vi "Dresden Edit Recipe(in).vi"() -> ()   [LabVIEW 2009] (continued)
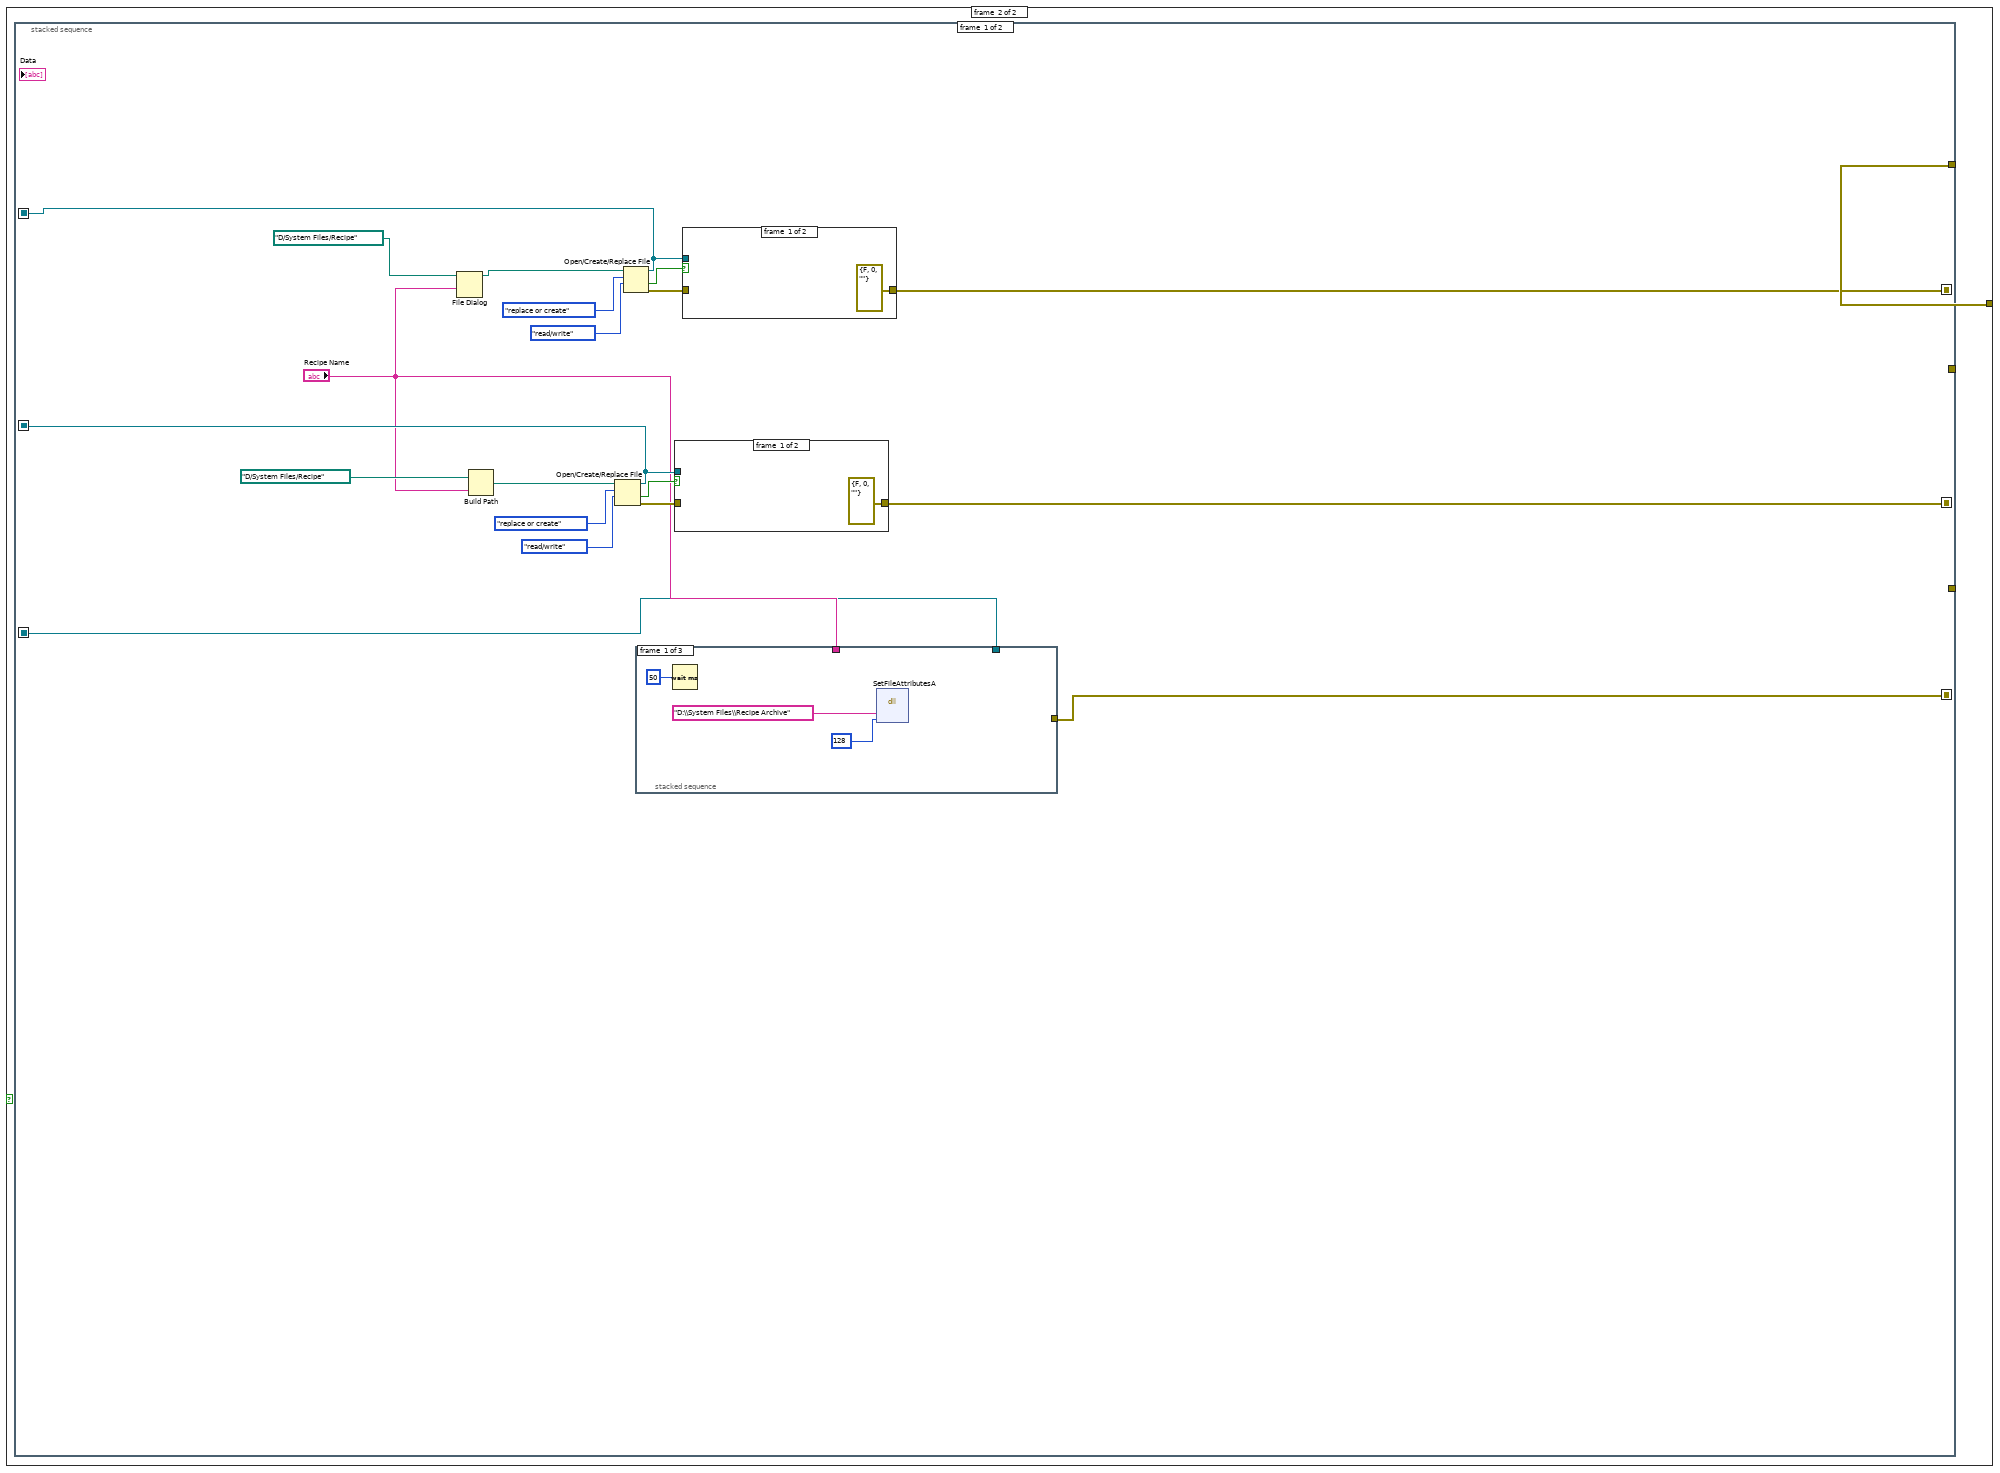
[diagram p2: hidden frame]
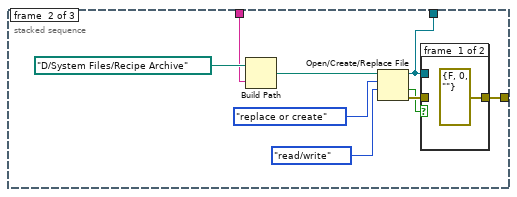
[diagram p3: hidden frame]
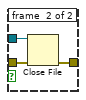
[diagram p4: hidden frame]
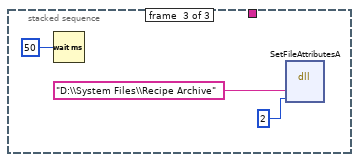
[diagram p5: hidden frame]
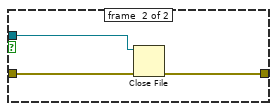
[diagram p6: hidden frame]
                }
                frame #1 {
                }
              }
              n2527 = Format Into String(format string="%s%s%s%s%s", "\r", "Ramp Down Time(s):" ("input 2"), w3329, w3329, w3327) -> (resulting string=w3326:string)  [unwired: 2 in, 1 out]
            }
            frame #89 {
              w3337 = "\r"
              w3338 = "\t"
              n2528 = local read "R Single RF Ramp down Time"() -> (w3336:dbl)
              n2529 = Format Into String(format string="%s%s%s%s%d%s%s", "\r", "Ramp Down Time(s):" ("input 2"), w3338, w3338, w3336, w3337, w3337) -> (resulting string=w3335:string)  [unwired: 2 in, 1 out]
            }
            frame #90 {
              w3343 = "\r"
              n2530 = Format Into String(format string="%s%s%s", "Multilayer Recipe Parameters" ("input 1"), w3343, w3343) -> (resulting string=w3342:string)  [unwired: 2 in, 1 out]
            }
            frame #91 {
              n2531 = Format Into String(format string="%s%s", "DC Parameters" ("input 1"), "\r") -> (resulting string=w3346:string)  [unwired: 2 in, 1 out]
            }
            frame #92 {
              w3352 = "\t"
              n2532 = local read "R Cmb Ch2 Target material"() -> (w3351:string)
              n2533 = Format Into String(format string="%s%s%s%s%s", "\r", "Target Material:" ("input 2"), w3352, w3352, w3351) -> (resulting string=w3350:string)  [unwired: 2 in, 1 out]
            }
            frame #93 {
              w3358 = "\t"
              n2534 = local read "R_Cmb_Ch2_Web_speed"() -> (w3357:dbl)
              n2535 = Format Into String(format string="%s%s%s%s%d", "\r", "Web Speed(cm/sec):" ("input 2"), w3358, w3358, w3357) -> (resulting string=w3356:string)  [unwired: 2 in, 1 out]
            }
            frame #94 {
              w3364 = "\t"
              n2536 = local read "R Cmb Ch3 Target material"() -> (w3363:string)
              n2537 = Format Into String(format string="%s%s%s%s%s", "\r", "Target Material:" ("input 2"), w3364, w3364, w3363) -> (resulting string=w3362:string)  [unwired: 2 in, 1 out]
            }
            frame #95 {
              w3370 = "\t"
              n2538 = local read "R_Cmb_Ch3_Web_speed"() -> (w3369:dbl)
              n2539 = Format Into String(format string="%s%s%s%s%d", "\r", "Web Speed(cm/sec):" ("input 2"), w3370, w3370, w3369) -> (resulting string=w3368:string)  [unwired: 2 in, 1 out]
            }
            frame #96 {
              w3377 = "\t"
              n2540 = local read "R Cmb Step1 Coating Power Active"() -> (w3375:bool)
              n2541 = case shown="False" w3375 {
                tunnel: ["Deactive" ("input 4") "Active" ("input 4")] -> w3376
                frame #0 {
                }
                frame #1 {
                }
              }
              n2542 = Format Into String(format string="%s%s%s%s%s%s", "\r", "Region 1:" ("input 2"), w3377, w3377, w3377, w3376) -> (resulting string=w3374:string)  [unwired: 2 in, 1 out]
            }
            frame #97 {
              w3388 = "\t"
              n2543 = local read "R Cmb Ch2 Step1 Coating Power"() -> (w3384:dbl)
              n2544 = Format Into String(format string="%s%s%s%s%s%d", "\r", "CH2-Power(W):" ("input 2"), w3388, w3388, w3388, w3384) -> (resulting string=w3383:string)  [unwired: 2 in, 1 out]
            }
            frame #98 {
              w3391 = "\t"
              n2545 = local read "R Cmb Ch3 Step1 Coating Power"() -> (w3390:dbl)
              n2546 = Format Into String(format string="%s%s%s%s%s%d", "\r", "CH3-Power(W):" ("input 2"), w3391, w3391, w3391, w3390) -> (resulting string=w3389:string)  [unwired: 2 in, 1 out]
            }
            frame #99 {
              w3397 = "\t"
              n2547 = local read "R Cmb Interval length 1"() -> (w3396:dbl)
              n2548 = Format Into String(format string="%s%s%s%s%d", "\r", "Interval Length(m):" ("input 2"), w3397, w3397, w3396) -> (resulting string=w3395:string)  [unwired: 2 in, 1 out]
            }
            frame #100 {
              w3403 = "\t"
              n2549 = local read "R Cmb Step2 Coating Power Active"() -> (w3401:bool)
              n2550 = case shown="True" w3401 {
                tunnel: ["Deactive" ("input 4") "Active" ("input 4")] -> w3404
                frame #0 {
                }
                frame #1 {
                }
              }
              n2551 = Format Into String(format string="%s%s%s%s%s%s", "\r", "Region 2:" ("input 2"), w3403, w3403, w3403, w3404) -> (resulting string=w3402:string)  [unwired: 2 in, 1 out]
            }
            frame #101 {
              w3415 = "\t"
              n2552 = local read "R Cmb Ch2 Step2 Coating Power"() -> (w3410:dbl)
              n2553 = Format Into String(format string="%s%s%s%s%s%d", "\r", "CH2-Power(W):" ("input 2"), w3415, w3415, w3415, w3410) -> (resulting string=w3411:string)  [unwired: 2 in, 1 out]
            }
            frame #102 {
              w3421 = "\t"
              n2554 = local read "R Cmb Ch3 Step2 Coating Power"() -> (w3416:dbl)
              n2555 = Format Into String(format string="%s%s%s%s%s%d", "\r", "CH3-Power(W):" ("input 2"), w3421, w3421, w3421, w3416) -> (resulting string=w3418:string)  [unwired: 2 in, 1 out]
            }
            frame #103 {
              w3424 = "\t"
              n2556 = local read "R Cmb Interval length 2"() -> (w3423:dbl)
              n2557 = Format Into String(format string="%s%s%s%s%d", "\r", "Interval Length(m):" ("input 2"), w3424, w3424, w3423) -> (resulting string=w3422:string)  [unwired: 2 in, 1 out]
            }
            frame #104 {
              w3430 = "\t"
              n2558 = local read "R Cmb Step3 Coating Power Active"() -> (w3429:bool)
              n2559 = case shown="False" w3429 {
                tunnel: ["Deactive" ("input 4") "Active" ("input 4")] -> w3431
                frame #0 {
                }
                frame #1 {
                }
              }
              n2560 = Format Into String(format string="%s%s%s%s%s%s", "\r", "Region 3:" ("input 2"), w3430, w3430, w3430, w3431) -> (resulting string=w3428:string)  [unwired: 2 in, 1 out]
            }
            frame #105 {
              w3442 = "\t"
              n2561 = local read "R Cmb Ch2 Step3 Coating Power"() -> (w3437:dbl)
              n2562 = Format Into String(format string="%s%s%s%s%s%d", "\r", "CH2-Power(W):" ("input 2"), w3442, w3442, w3442, w3437) -> (resulting string=w3439:string)  [unwired: 2 in, 1 out]
            }
            frame #106 {
              w3448 = "\t"
              n2563 = local read "R Cmb Ch3 Step3 Coating Power"() -> (w3443:dbl)
              n2564 = Format Into String(format string="%s%s%s%s%s%d", "\r", "CH3-Power(W):" ("input 2"), w3448, w3448, w3448, w3443) -> (resulting string=w3445:string)  [unwired: 2 in, 1 out]
            }
            frame #107 {
              w3451 = "\t"
              n2565 = local read "R Cmb Interval length 3"() -> (w3450:dbl)
              n2566 = Format Into String(format string="%s%s%s%s%d", "\r", "Interval Length(m):" ("input 2"), w3451, w3451, w3450) -> (resulting string=w3449:string)  [unwired: 2 in, 1 out]
            }
            frame #108 {
              w3457 = "\t"
              n2567 = local read "R Cmb Step4 Coating Power Active"() -> (w3456:bool)
              n2568 = case shown="False" w3456 {
                tunnel: ["Deactive" ("input 4") "Active" ("input 4")] -> w3458
                frame #0 {
                }
                frame #1 {
                }
              }
              n2569 = Format Into String(format string="%s%s%s%s%s%s", "\r", "Region 4:" ("input 2"), w3457, w3457, w3457, w3458) -> (resulting string=w3455:string)  [unwired: 2 in, 1 out]
            }
            frame #109 {
              w3469 = "\t"
              n2570 = local read "R Cmb Ch2 Step4 Coating Power"() -> (w3465:dbl)
              n2571 = Format Into String(format string="%s%s%s%s%s%d", "\r", "CH2-Power(W):" ("input 2"), w3469, w3469, w3469, w3465) -> (resulting string=w3466:string)  [unwired: 2 in, 1 out]
            }
            frame #110 {
              w3475 = "\t"
              n2572 = local read "R Cmb Ch3 Step4 Coating Power"() -> (w3471:dbl)
              n2573 = Format Into String(format string="%s%s%s%s%s%d", "\r", "CH3-Power(W):" ("input 2"), w3475, w3475, w3475, w3471) -> (resulting string=w3472:string)  [unwired: 2 in, 1 out]
            }
            frame #111 {
              w3478 = "\t"
              n2574 = local read "R Cmb Interval length 4"() -> (w3477:dbl)
              n2575 = Format Into String(format string="%s%s%s%s%d", "\r", "Interval Length(m):" ("input 2"), w3478, w3478, w3477) -> (resulting string=w3476:string)  [unwired: 2 in, 1 out]
            }
            frame #112 {
              w3484 = "\t"
              n2576 = local read "R Cmb Step5 Coating Power Active"() -> (w3483:bool)
              n2577 = case shown="False" w3483 {
                tunnel: ["Deactive" ("input 4") "Active" ("input 4")] -> w3485
                frame #0 {
                }
                frame #1 {
                }
              }
              n2578 = Format Into String(format string="%s%s%s%s%s%s", "\r", "Region 5:" ("input 2"), w3484, w3484, w3484, w3485) -> (resulting string=w3482:string)  [unwired: 2 in, 1 out]
            }
            frame #113 {
              w3496 = "\t"
              n2579 = local read "R Cmb Ch2 Step5 Coating Power"() -> (w3491:dbl)
              n2580 = Format Into String(format string="%s%s%s%s%s%d", "\r", "CH2-Power(W):" ("input 2"), w3496, w3496, w3496, w3491) -> (resulting string=w3493:string)  [unwired: 2 in, 1 out]
            }
            frame #114 {
              w3502 = "\t"
              n2581 = local read "R Cmb Ch3 Step5 Coating Power"() -> (w3497:dbl)
              n2582 = Format Into String(format string="%s%s%s%s%s%d", "\r", "CH3-Power(W):" ("input 2"), w3502, w3502, w3502, w3497) -> (resulting string=w3499:string)  [unwired: 2 in, 1 out]
            }
            frame #115 {
              w3505 = "\t"
              n2583 = local read "R Cmb Interval length 5"() -> (w3504:dbl)
              n2584 = Format Into String(format string="%s%s%s%s%d", "\r", "Interval Length(m):" ("input 2"), w3505, w3505, w3504) -> (resulting string=w3503:string)  [unwired: 2 in, 1 out]
            }
            frame #116 {
              w3511 = "\t"
              n2585 = local read "R Cmb Step6 Coating Power Active"() -> (w3510:bool)
              n2586 = case shown="False" w3510 {
                tunnel: ["Deactive" ("input 4") "Active" ("input 4")] -> w3512
                frame #0 {
                }
                frame #1 {
                }
              }
              n2587 = Format Into String(format string="%s%s%s%s%s%s", "\r", "Region 6:" ("input 2"), w3511, w3511, w3511, w3512) -> (resulting string=w3509:string)  [unwired: 2 in, 1 out]
            }
            frame #117 {
              w3520 = "\t"
              n2588 = local read "R Cmb Ch2 Step6 Coating Power"() -> (w3518:dbl)
              n2589 = Format Into String(format string="%s%s%s%s%s%d", "\r", "CH2-Power(W):" ("input 2"), w3520, w3520, w3520, w3518) -> (resulting string=w3521:string)  [unwired: 2 in, 1 out]
            }
            frame #118 {
              w3529 = "\t"
              n2590 = local read "R Cmb Ch3 Step6 Coating Power"() -> (w3524:dbl)
              n2591 = Format Into String(format string="%s%s%s%s%s%d", "\r", "CH3-Power(W):" ("input 2"), w3529, w3529, w3529, w3524) -> (resulting string=w3526:string)  [unwired: 2 in, 1 out]
            }
            frame #119 {
              w3532 = "\t"
              n2592 = local read "R Cmb Interval length 6"() -> (w3531:dbl)
              n2593 = Format Into String(format string="%s%s%s%s%d", "\r", "Interval Length(m):" ("input 2"), w3532, w3532, w3531) -> (resulting string=w3530:string)  [unwired: 2 in, 1 out]
            }
            frame #120 {
              w3538 = "\t"
              n2594 = local read "R Cmb Step7 Coating Power Active"() -> (w3537:bool)
              n2595 = case shown="False" w3537 {
                tunnel: ["Deactive" ("input 4") "Active" ("input 4")] -> w3539
                frame #0 {
                }
                frame #1 {
                }
              }
              n2596 = Format Into String(format string="%s%s%s%s%s%s", "\r", "Region 7:" ("input 2"), w3538, w3538, w3538, w3539) -> (resulting string=w3536:string)  [unwired: 2 in, 1 out]
            }
            frame #121 {
              w3550 = "\t"
              n2597 = local read "R Cmb Ch2 Step7 Coating Power"() -> (w3546:dbl)
              n2598 = Format Into String(format string="%s%s%s%s%s%d", "\r", "CH2-Power(W):" ("input 2"), w3550, w3550, w3550, w3546) -> (resulting string=w3547:string)  [unwired: 2 in, 1 out]
            }
            frame #122 {
              w3556 = "\t"
              n2599 = local read "R Cmb Ch3 Step7 Coating Power"() -> (w3551:dbl)
              n2600 = Format Into String(format string="%s%s%s%s%s%d", "\r", "CH3-Power(W):" ("input 2"), w3556, w3556, w3556, w3551) -> (resulting string=w3553:string)  [unwired: 2 in, 1 out]
            }
            frame #123 {
              w3559 = "\t"
              n2601 = local read "R Cmb Interval length 7"() -> (w3558:dbl)
              n2602 = Format Into String(format string="%s%s%s%s%d", "\r", "Interval Length(m):" ("input 2"), w3559, w3559, w3558) -> (resulting string=w3557:string)  [unwired: 2 in, 1 out]
            }
            frame #124 {
              w3565 = "\t"
              n2603 = local read "R Cmb Step8 Coating Power Active"() -> (w3564:bool)
              n2604 = case shown="False" w3564 {
                tunnel: ["Deactive" ("input 4") "Active" ("input 4")] -> w3566
                frame #0 {
                }
                frame #1 {
                }
              }
              n2605 = Format Into String(format string="%s%s%s%s%s%s", "\r", "Region 8:" ("input 2"), w3565, w3565, w3565, w3566) -> (resulting string=w3563:string)  [unwired: 2 in, 1 out]
            }
            frame #125 {
              w3577 = "\t"
              n2606 = local read "R Cmb Ch3 Step8 Coating Power"() -> (w3572:dbl)
              n2607 = Format Into String(format string="%s%s%s%s%s%d", "\r", "CH2-Power(W):" ("input 2"), w3577, w3577, w3577, w3572) -> (resulting string=w3574:string)  [unwired: 2 in, 1 out]
            }
            frame #126 {
              w3583 = "\t"
              n2608 = local read "R Cmb Ch3 Step8 Coating Power"() -> (w3579:dbl)
              n2609 = Format Into String(format string="%s%s%s%s%s%d", "\r", "CH3-Power(W):" ("input 2"), w3583, w3583, w3583, w3579) -> (resulting string=w3580:string)  [unwired: 2 in, 1 out]
            }
            frame #127 {
              w3586 = "\t"
              n2610 = local read "R Cmb Interval length 8"() -> (w3585:dbl)
              n2611 = Format Into String(format string="%s%s%s%s%d", "\r", "Interval Length(m):" ("input 2"), w3586, w3586, w3585) -> (resulting string=w3584:string)  [unwired: 2 in, 1 out]
            }
            frame #128 {
              w3592 = "\t"
              n2612 = local read "R Cmb Step9 Coating Power Active"() -> (w3591:bool)
              n2613 = case shown="False" w3591 {
                tunnel: ["Deactive" ("input 4") "Active" ("input 4")] -> w3593
                frame #0 {
                }
                frame #1 {
                }
              }
              n2614 = Format Into String(format string="%s%s%s%s%s%s", "\r", "Region 9:" ("input 2"), w3592, w3592, w3592, w3593) -> (resulting string=w3590:string)  [unwired: 2 in, 1 out]
            }
            frame #129 {
              w3604 = "\t"
              n2615 = local read "R Cmb Ch2 Step9 Coating Power"() -> (w3600:dbl)
              n2616 = Format Into String(format string="%s%s%s%s%s%d", "\r", "CH2-Power(W):" ("input 2"), w3604, w3604, w3604, w3600) -> (resulting string=w3601:string)  [unwired: 2 in, 1 out]
            }
            frame #130 {
              w3610 = "\t"
              n2617 = local read "R Cmb Ch3 Step9 Coating Power"() -> (w3605:dbl)
              n2618 = Format Into String(format string="%s%s%s%s%s%d", "\r", "CH3-Power(W):" ("input 2"), w3610, w3610, w3610, w3605) -> (resulting string=w3607:string)  [unwired: 2 in, 1 out]
            }
            frame #131 {
              w3613 = "\t"
              n2619 = local read "R Cmb Interval length 9"() -> (w3612:dbl)
              n2620 = Format Into String(format string="%s%s%s%s%d", "\r", "Interval Length(m):" ("input 2"), w3613, w3613, w3612) -> (resulting string=w3611:string)  [unwired: 2 in, 1 out]
            }
            frame #132 {
              w3619 = "\t"
              n2621 = local read "R Cmb Step10 Coating Power Active"() -> (w3618:bool)
              n2622 = case shown="False" w3618 {
                tunnel: ["Deactive" ("input 4") "Active" ("input 4")] -> w3620
                frame #0 {
                }
                frame #1 {
                }
              }
              n2623 = Format Into String(format string="%s%s%s%s%s%s", "\r", "Region 10:" ("input 2"), w3619, w3619, w3619, w3620) -> (resulting string=w3617:string)  [unwired: 2 in, 1 out]
            }
            frame #133 {
              w3631 = "\t"
              n2624 = local read "R Cmb Ch2 Step10 Coating Power"() -> (w3626:dbl)
              n2625 = Format Into String(format string="%s%s%s%s%s%d", "\r", "CH2-Power(W):" ("input 2"), w3631, w3631, w3631, w3626) -> (resulting string=w3628:string)  [unwired: 2 in, 1 out]
            }
            frame #134 {
              w3637 = "\t"
              n2626 = local read "R Cmb Ch3 Step10 Coating Power"() -> (w3633:dbl)
              n2627 = Format Into String(format string="%s%s%s%s%s%d", "\r", "CH3-Power(W):" ("input 2"), w3637, w3637, w3637, w3633) -> (resulting string=w3634:string)  [unwired: 2 in, 1 out]
            }
            frame #135 {
              w3641 = "\t"
              n2628 = local read "R Cmb Interval length 10"() -> (w3640:dbl)
              n2629 = Format Into String(format string="%s%s%s%s%d%s", "\r", "Interval Length(m):" ("input 2"), w3641, w3641, w3640, "\r") -> (resulting string=w3639:string)  [unwired: 2 in, 1 out]
            }
            frame #136 {
              w3648 = "\t"
              n2630 = local read "R_First_stop_selection"() -> (w3647:enum32{"Chamber II", "Chamber III"})
              n2631 = case shown="\"Chamber III\"" w3647 {
                tunnel: ["Chamber II" ("string") "Chamber III" ("string")] -> w3645
                frame #0 {
                }
                frame #1 {
                }
              }
              n2632 = Format Into String(format string="%s%s%s%s", "First Stop Selection:" ("input 1"), w3648, w3648, w3645) -> (resulting string=w3646:string)  [unwired: 2 in, 1 out]
            }
            frame #137 {
              w3655 = "\r"
              w3656 = "\t"
              n2633 = local read "R Cmb Number of cycle"() -> (w3654:dbl)
              n2634 = Format Into String(format string="%s%s%s%s%d%s%s", "\r", "Number of cycle:" ("input 2"), w3656, w3656, w3654, w3655, w3655) -> (resulting string=w3653:string)  [unwired: 2 in, 1 out]
            }
            frame #138 {
              w3662 = "\t"
              n2635 = Format Into String(format string="%s%s%s%s", "Pressure Control Parameters" ("input 1"), w3662, w3662, "\r") -> (resulting string=w3660:string)  [unwired: 2 in, 1 out]
            }
            frame #139 {
              w3667 = "\t"
              n2636 = local read "R Argon Flow sccm"() -> (w3666:dbl)
              n2637 = Format Into String(format string="%s%s%s%s%d", "\r", "Argon Flow(sccm) :" ("input 2"), w3667, w3667, w3666) -> (resulting string=w3665:string)  [unwired: 2 in, 1 out]
            }
            frame #140 {
              w3672 = "\r"
              w3674 = "\t"
              n2638 = local read "R Set Pressure mtorr"() -> (w3673:dbl)
              n2639 = Format Into String(format string="%s%s%s%s%.1f%s%s", "\r", "Set Pressure(mTorr):" ("input 2"), w3674, w3674, w3673, w3672, w3672) -> (resulting string=w3671:string)  [unwired: 2 in, 1 out]
            }
            frame #141 {
              w3680 = "\t"
              n2640 = Format Into String(format string="%s%s%s%s", "Thickness Monitor Parameters" ("input 1"), w3680, w3680, "\r") -> (resulting string=w3678:string)  [unwired: 2 in, 1 out]
            }
            frame #142 {
              w3686 = "\t"
              n2641 = local read "Thickness_Monitor_Active"() -> (w3683:bool)
              n2642 = case shown="False" w3683 {
                tunnel: ["Deactive" ("input 4") "Active" ("input 4")] -> w3684
                frame #0 {
                }
                frame #1 {
                }
              }
              n2643 = Format Into String(format string="%s%s%s%s%s", "\r", "Thickness Monitor:" ("input 2"), w3686, w3686, w3684) -> (resulting string=w3685:string)  [unwired: 2 in, 1 out]
            }
            frame #143 {
              n2644 = local read "R Material_density"() -> (w3693:dbl)
              n2645 = Format Into String(format string="%s%s%s%.2f", "\r", "Material Density(g/cm3) :" ("input 2"), "\t", w3693) -> (resulting string=w3692:string)  [unwired: 2 in, 1 out]
            }
            frame #144 {
              w3700 = "\t"
              n2646 = local read "R Z_factor"() -> (w3699:dbl)
              n2647 = Format Into String(format string="%s%s%s%s%s%.2f", "\r", "Z Factor:" ("input 2"), w3700, w3700, w3700, w3699) -> (resulting string=w3698:string)  [unwired: 2 in, 1 out]
            }
            frame #145 {
              w3706 = "\t"
              n2648 = local read "R Toooling_factor"() -> (w3705:dbl)
              n2649 = Format Into String(format string="%s%s%s%s%d", "\r", "Tooling Factor (%):" ("input 2"), w3706, w3706, w3705) -> (resulting string=w3704:string)  [unwired: 2 in, 1 out]
            }
          }
          n2650 = Concatenate Strings(w2706, w2705, w2704, w2703, w2702, w2701, w2700, w2699, w2698, w2697, w2696, w2695, w2694, w2693, w2692, w2691, w2690, w2689, w2688, w2687, w2686, w2685, w2684, w2683, w2682, w2681, w2680, w2679, w2678, w2677, w2676, w2675, w2674, w2673, w2672, w2671, w2670, w2669, w2668, w2667, w2666, w2665, w2664, w2663, w2662, w2661, w2660, w2659, w2658, w2657, w2656, w2655, w2654, w2653, w2652, w2651, w2650, w2649, w2648, w2647, w2646, w2645, w2644, w2643, w2642, w2641, w2640, w2639, w2638, w2637, w2636, w2635, w2634, w2633, w2632, w2631, w2630, w2629, w2628, w2627, w2626, w2625, w2624, w2623, w2622, w2621, w2620, w2619, w2618, w2617, w2616, w2615, w2614, w2613, w2612, w2611, w2610, w2609, w2608, w2607, w2606, w2605, w2604, w2603, w2602, w2601, w2600, w2599, w2598, w2597, w2596, w2595, w2594, w2593, w2592, w2591, w2590, w2589, w2588, w2587, w2586, w2585, w2584, w2583, w2582, w2581, w2580, w2579, w2578, w2577, w2576, w2575, w2574, w2573, w2572, w2571, w2570, w2569, w2568, w2567, w2566, w2565, w2564, w2563, w2562, w2561) -> (w2709:string)
          n2651 = Write to Text File(file (use dialog)=w2708, text=w2709, error in=w2711) -> (refnum out=w2707:refnum<file>, error out=w2712:errorcluster)  [unwired: 1 in, 1 out]
          n2652 = Write to Text File(file (use dialog)=w2720, text=w2709, error in=w2718) -> (refnum out=w2721:refnum<file>, error out=w2722:errorcluster)  [unwired: 1 in, 1 out]
          n2653 = Write to Text File(file (use dialog)=w2715, text=w2709, error in=w2714) -> (refnum out=w2716:refnum<file>, error out=w2717:errorcluster)  [unwired: 1 in, 1 out]
          n2654 = Close File(refnum=w2707, error in=w2712) -> (error out=w2710:errorcluster)  [unwired: 1 out]
          n2655 = Close File(refnum=w2721, error in=w2722) -> (error out=w2719:errorcluster)  [unwired: 1 out]
          n2656 = Close File(refnum=w2716, error in=w2717) -> (error out=w2713:errorcluster)  [unwired: 1 out]
        }
      }
    }
  }
  "error out" <- w2
  n2657 = Not(x=w1) -> (.not. x?=w3:bool)
  n2658 = property class="VI"("Front Panel Window:Open"=w3) -> ()  [unwired: 2 in, 2 out]
